vi "Autonomous Vars.vi"() -> ()   [LabVIEW 2020]
panel:
  in  "Setpoint Rotation":dbl
  in  "Setpoint Y":dbl
  in  "Setpoint X":dbl
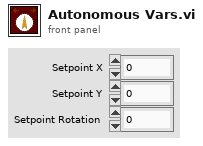
[diagram p1: front panel]
diagram:
